vi "Main.vi"() -> ()   [LabVIEW 2014, in "Manipulator.lvclass"]
uses:
  Manipulator.lvclass
  typedefs/Coordinates.ctl
  <vilib>/Analysis/Matrix/Datatypes/RealMatrix.ctl
  typedefs/CommandStructure.ctl
  <vilib>/Analysis/Matrix/NI_Matrix.lvlib
panel:
  in  "STOP":bool
  out "Message":string
  in  "Visualization":refnum<k7>(container) caption="Visualisation in 3D"
  in  "Tab":enum32{"Visualisation 3D", "Trajectory Builder"}(tab)
  in  "MethodOfCalculation":u16(ring) items=["Geometric Method", "Denavit-Hartenberg Convention"]
  in  "AddPoint":bool
  in  "Cluster":T1={"Theta 1 "=45.0, "Theta 2"=90.0, "Theta 3"=90.0, "Theta 4"=90.0} {"Theta 4" min=0.0 max=180.0 step=0.5; "Theta 3" min=0.0 max=180.0 step=0.5; "Theta 2" min=0.0 max=180.0 step=0.5; "Theta 1" min=0.0 max=90.0 step=0.5}
  in  "CoordinatesIN":T2={"X"=141.5, "Y"=141.5, "Z"=220.5} {"X" step=0.5; "Y" step=0.5; "Z" step=0.5}
  out "ArrayOfNames\nOfPoints":string[](array[string])=["Point 1"]
  in  "NumberOfPoints":dbl=1.0 min=1.0 max=10.0 step=1.0
  in  "MatrixOfPoints":T3
  in  "Generate":bool
  # "CARTESIAN"
  # "JOINTS"
  # "PLEASE CHOOSE HOW MANY POINTS \nYOU WANT IN YOUR PATH"
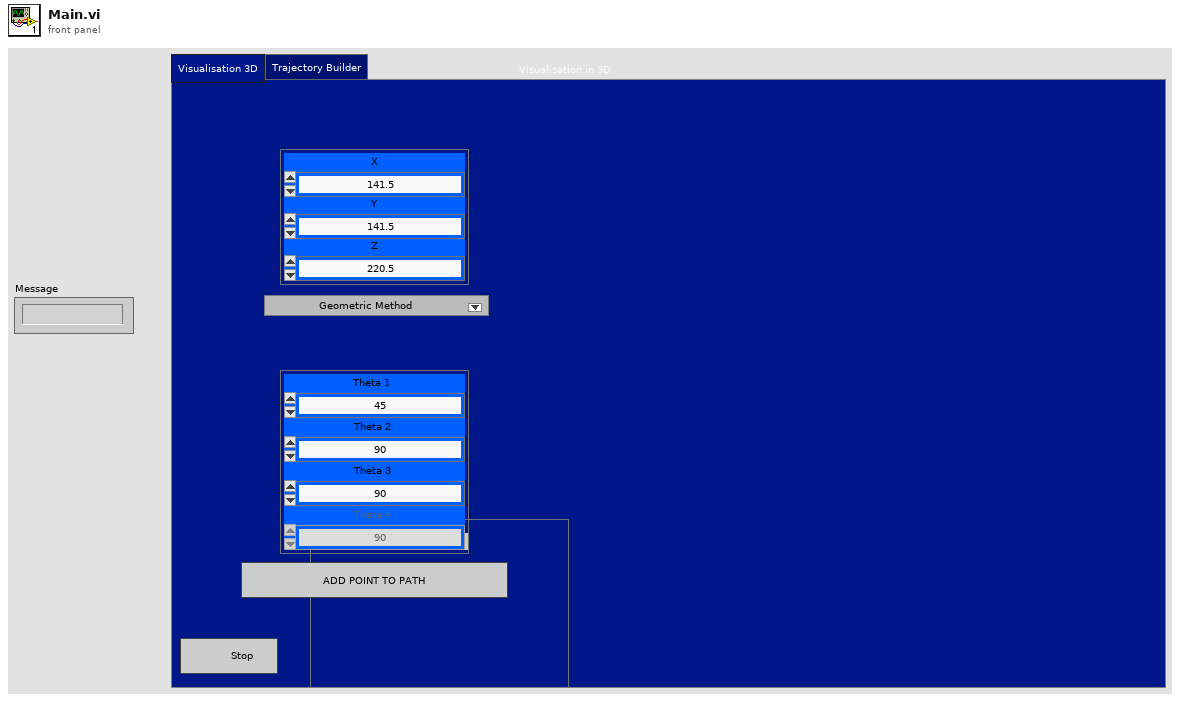
[diagram p1: front panel]
types:
  T1 = cluster{"Theta 1 ":dbl, "Theta 2":dbl, "Theta 3":dbl, "Theta 4":dbl}
  T2 = typedef "Manipulator.lvclass/Coordinates.ctl" = cluster{"X":dbl, "Y":dbl, "Z":dbl}
  T3 = typedef "NI_Matrix.lvlib/RealMatrix.ctl" = dbl[][]
  T4 = typedef "Manipulator.lvclass/CommandStructure.ctl" = cluster{"Command":string, "Data":variant}
  T5 = cluster{"Cluster":cluster{"Theta 1 ":dbl, "Theta 2":dbl, "Theta 3":dbl, "Theta 4":dbl}, "Cluster 2":cluster{"Theta 1 ":dbl, "Theta 2":dbl, "Theta 3":dbl, "Theta 4":dbl}}
  T6 = cluster{"NewVal":cluster{"X":dbl, "Y":dbl, "Z":dbl}, "OldVal":cluster{"X":dbl, "Y":dbl, "Z":dbl}}
  T7 = cluster{"Theta 1 ":dbl, "Theta 2":dbl, "Theta 3":dbl}
  T8 = cluster{"Numeric Control":dbl, "Numeric Control":dbl, "Numeric Control":dbl}
  T9 = cluster{"THETA_1":dbl, "THETA_2":dbl, "THETA_3":dbl, "THETA_4":dbl, "THETA_5":dbl, "THETA_6":dbl, "THETA_7":dbl, "THETA_8":dbl, "THETA_9":dbl, "THETA_10":dbl}[]
  T10 = cluster{"THETA_1":dbl, "THETA_2":dbl, "THETA_3":dbl, "THETA_4":dbl, "THETA_5":dbl, "THETA_6":dbl, "THETA_7":dbl, "THETA_8":dbl, "THETA_9":dbl, "THETA_10":dbl}
  T11 = cluster{"THETA_1":dbl, "THETA_2":dbl, "THETA_6":dbl, "THETA_4":dbl}
  T12 = cluster{"Numeric Control":dbl, "Numeric Control":dbl, "Numeric Control":dbl, "Numeric Control":dbl}
  T13 = cluster{"THETA_1":dbl, "THETA_2":dbl, "THETA_6":dbl, "THETA_4":dbl}[]
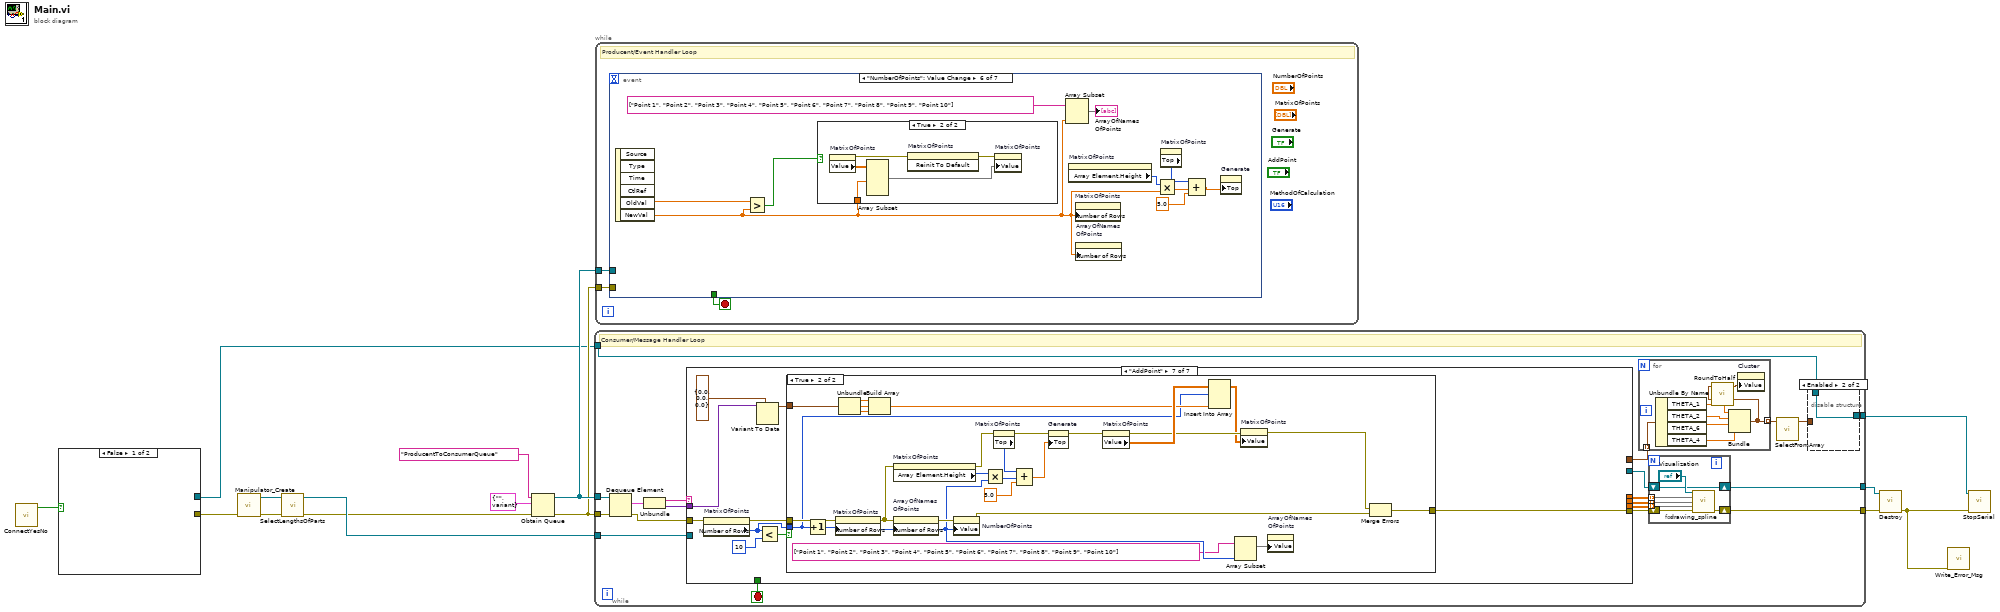
[diagram p0: block diagram]
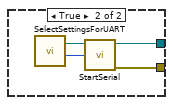
[diagram p2: hidden frame]
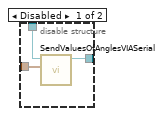
[diagram p3: hidden frame]
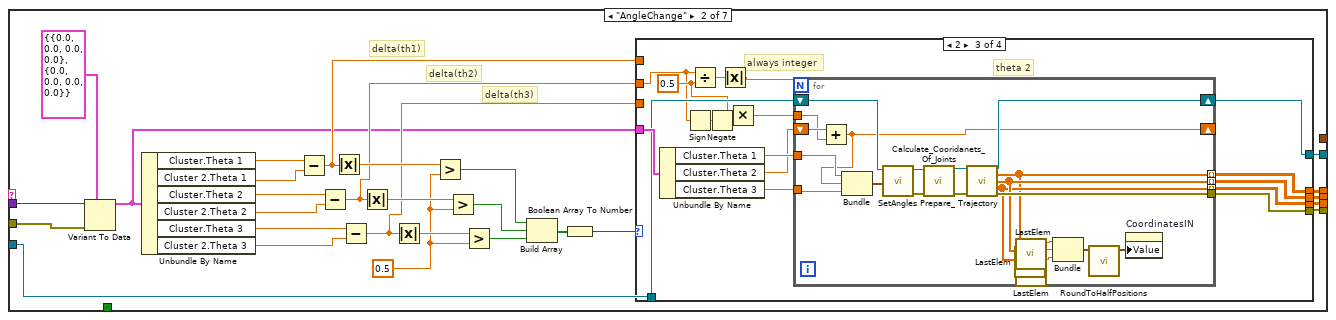
[diagram p5: hidden frame]
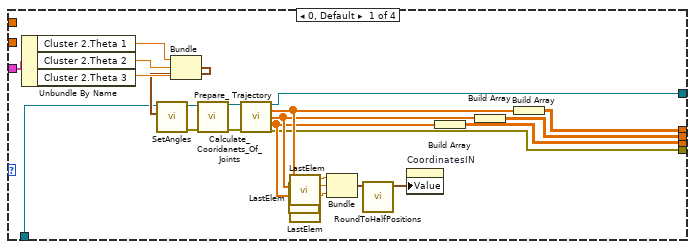
[diagram p6: hidden frame]
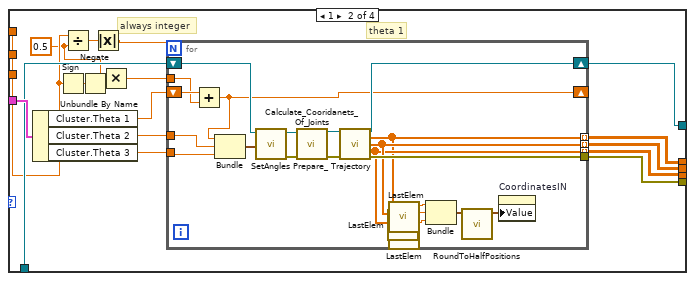
[diagram p7: hidden frame]
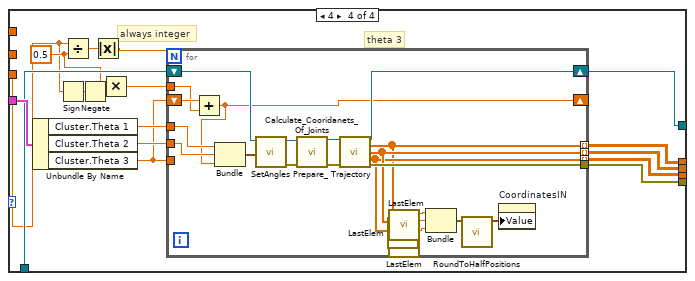
[diagram p8: hidden frame]
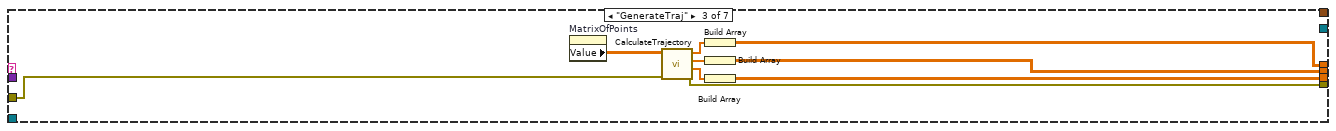
[diagram p9: hidden frame]
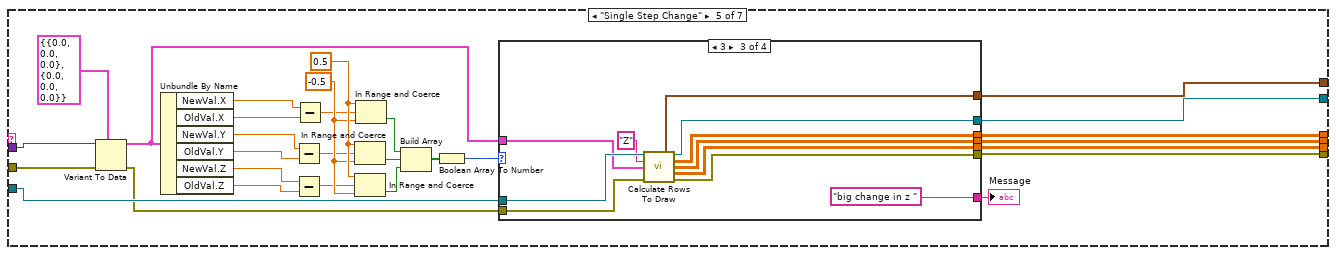
[diagram p11: hidden frame]
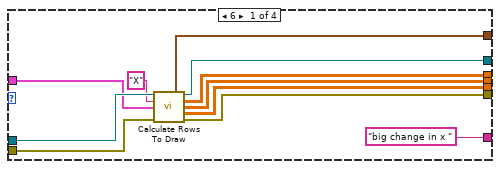
[diagram p12: hidden frame]
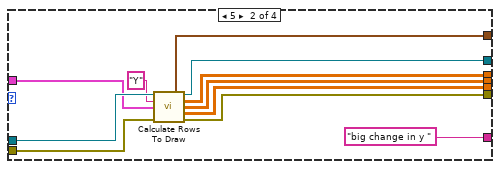
[diagram p13: hidden frame]
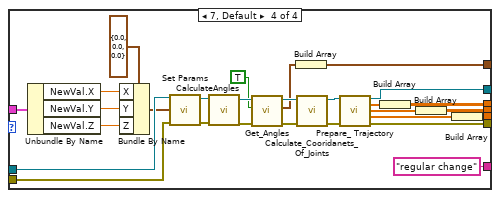
[diagram p14: hidden frame]
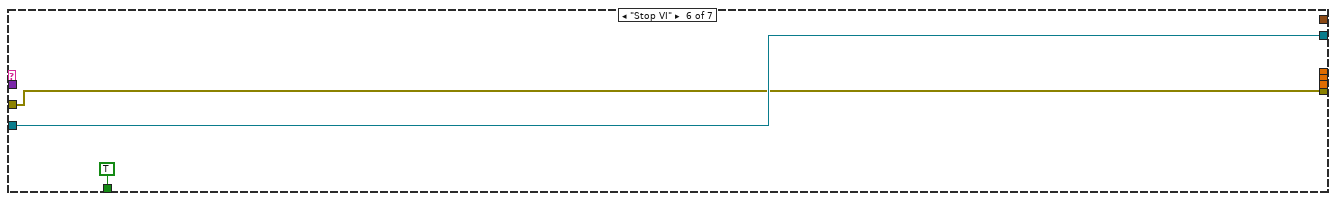
[diagram p15: hidden frame]
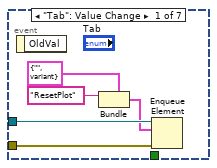
[diagram p17: hidden frame]
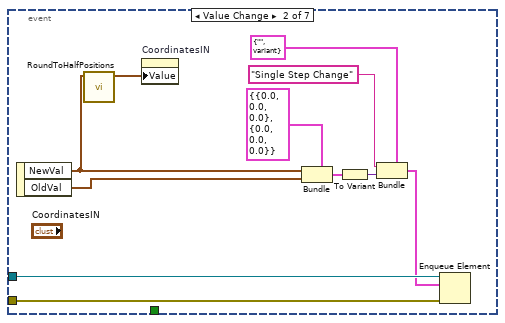
[diagram p18: hidden frame]
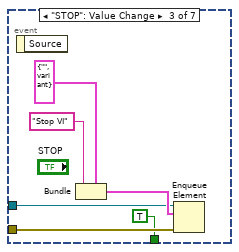
[diagram p19: hidden frame]
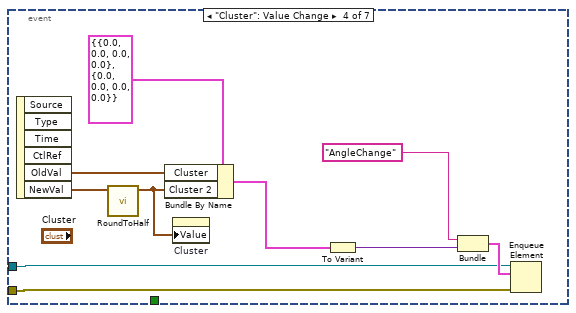
[diagram p20: hidden frame]
diagram:
  n1 = call "ConnectYesNo"() -> ("connect?"=w1:bool)  [unwired: 11 in]
  n2 = case shown="False" w1 {
    tunnel: [_ w19] -> w5
    tunnel: [_ w18] -> w4
    frame False {
    }
    frame True {
      n3 = call "SelectSettingsForUART.vi"() -> ("BaundRate"=w16:u32, "COMPort"=w17:refnum<visa-resource-name>)  [unwired: 10 in]
      n4 = call "StartSerial.vi"("baud rate"=w16, "VISA Refnum in"=w17) -> ("error out"=w19:errorcluster, "VISA Refnum out"=w18:refnum<visa-resource-name>)  [unwired: 8 in]
    }
  }
  n5 = call "Manipulator_Create.vi"("error in (no error)"=w5) -> ("error out"=w10:errorcluster, "reference out"=w12:refnum<class "Manipulator.lvclass">)  [unwired: 9 in]
  n6 = call-dynamic "SelectLengthsOfParts.vi"("error in (no error)"=w10, "reference in"=w12) -> ("error out"=w9:errorcluster, "reference out"=w11:refnum<class "Manipulator.lvclass">)  [unwired: 8 in]
  n7 = Obtain Queue(name (unnamed)="ProducentToConsumerQueue", element data type=T4 {"Command"="", "Data"=variant}, error in (no error)=w9) -> (queue out=w15:refnum<queue>, error out=w14:errorcluster)  [unwired: 2 in, 1 out]
  n8 = while {
    tunnel: w15 -> [w39]
    tunnel: w14 -> [w38]
    tunnel: w11 -> [w33]
    tunnel: [w30] -> w13
    tunnel: [w31] -> w6
    tunnel: w4 -> [w23]
    tunnel: [w22] -> w3
    stop <- w32 stop-if-true
    # "Consumer/Message Handler Loop"
    n9 = Dequeue Element(queue=w39, error in (no error)=w38) -> (element=w37:T4, error out=w34:errorcluster)  [unwired: 1 in, 2 out]
    n10 = Unbundle(w37) -> ("Command"=w36:string, "Data"=w35:variant)
    n11 = case shown="\"AddPoint\"" w36 {
      tunnel: w35 -> [_ w86 _ _ w260 _ w330]
      tunnel: [_ _ _ _ _ TRUE _] -> w32
      tunnel: w34 -> [w58 w85 w231 w233 w262 w324 w335]
      tunnel: w33 -> [_ w64 _ _ w242 w325 _]
      tunnel: [_ w63 _ _ w239 w325 _] -> w29
      tunnel: [w58 w62 w230 w233 w235 w324 w327] -> w28
      tunnel: [_ w61 w228 _ w238 _ _] -> w27
      tunnel: [_ w59 w226 _ w237 _ _] -> w26
      tunnel: [_ w60 w224 _ w236 _ _] -> w25
      tunnel: [_ _ _ _ w234 _ _] -> w24
      frame Default {
      }
      frame "AngleChange" {
        w75 = 0.5 ("y")
        # "delta(th3)"
        # "delta(th2)"
        # "delta(th1)"
        n12 = Variant To Data(error in=w85, type=T5 {"Cluster"={"Theta 1 "=0.0, "Theta 2"=0.0, "Theta 3"=0.0, "Theta 4"=0.0}, "Cluster 2"={"Theta 1 "=0.0, "Theta 2"=0.0, "Theta 3"=0.0, "Theta 4"=0.0}} ("input cluster"), Variant=w86) -> (data=w65:T5)  [unwired: 1 out]
        n13 = Unbundle By Name(w65) -> ("Cluster.Theta 1"=w66:dbl, "Cluster 2.Theta 1"=w83:dbl, "Cluster.Theta 2"=w82:dbl, "Cluster 2.Theta 2"=w81:dbl, "Cluster.Theta 3"=w80:dbl, "Cluster 2.Theta 3"=w79:dbl)
        n14 = Subtract(x=w66, y=w83) -> (x-y=w69:dbl)
        n15 = Subtract(x=w82, y=w81) -> (x-y=w67:dbl)
        n16 = Absolute Value(x=w69) -> (abs(x)=w78:dbl)
        n17 = Subtract(x=w80, y=w79) -> (x-y=w68:dbl)
        n18 = Absolute Value(x=w67) -> (abs(x)=w76:dbl)
        n19 = Absolute Value(x=w68) -> (abs(x)=w77:dbl)
        n20 = Greater?(x=w78, y=w75) -> (0:w74:bool)
        n21 = Greater?(x=w76, y=w75) -> (0:w73:bool)
        n22 = Greater?(x=w77, y=w75) -> (0:w72:bool)
        n23 = Build Array(w74, w73, w72) -> (w71:bool[])
        n24 = Boolean Array To Number(Boolean array=w71) -> (number=w70:u32)
        n25 = case shown="2" w70 {
          tunnel: w69 -> [_ w115 _ _]
          tunnel: w67 -> [_ _ w148 _]
          tunnel: w68 -> [_ _ _ w186]
          tunnel: w65 -> [w93 w126 w164 w202]
          tunnel: w64 -> [w88 w125 w163 w201]
          tunnel: [w87 w124 w162 w200] -> w63
          tunnel: [w94 w123 w161 w199] -> w62
          tunnel: [w99 w122 w160 w198] -> w61
          tunnel: [w95 w120 w158 w196] -> w60
          tunnel: [w97 w121 w159 w197] -> w59
          frame 0, Default {
            n26 = Unbundle By Name(w93) -> ("Cluster 2.Theta 1"=w92:dbl, "Cluster 2.Theta 2"=w91:dbl, "Cluster 2.Theta 3"=w90:dbl)
            n27 = Bundle("Theta 1"=w92, "Theta 2"=w91, "Theta 3"=w90) -> (w89:T7)  [unwired: 1 in]
            n28 = call-dynamic "SetAngles.vi"("Angles"=w89, "reference in"=w88) -> ("error out"=w106:errorcluster, "reference out"=w107:refnum<class "Manipulator.lvclass">)  [unwired: 8 in]
            n29 = call-dynamic "Calculate_Cooridanets_Of_Joints.vi"("error in (no error)"=w106, "reference in"=w107) -> ("error out"=w108:errorcluster, "reference out"=w109:refnum<class "Manipulator.lvclass">)  [unwired: 8 in]
            n30 = call-dynamic "Prepare_ Trajectory.vi"("reference in"=w109, "error in (no error)"=w108) -> ("reference out"=w87:refnum<class "Manipulator.lvclass">, "X"=w100:dbl[], "Y"=w98:dbl[], "Z"=w96:dbl[], "error out"=w94:errorcluster)  [unwired: 9 in]
            n31 = call "LastElem.vi"("X"=w98) -> ("Numeric Control"=w104:dbl)  [unwired: 10 in]
            n32 = call "LastElem.vi"("X"=w100) -> ("Numeric Control"=w105:dbl)  [unwired: 10 in]
            n33 = call "LastElem.vi"("X"=w96) -> ("Numeric Control"=w103:dbl)  [unwired: 10 in]
            n34 = Bundle("Numeric Control"=w105, "Numeric Control"=w104, "Numeric Control"=w103) -> (w102:T8)  [unwired: 1 in]
            n35 = call "RoundToHalfPositions.vi"("input cluster"=w102) -> ("output cluster"=w101:T8)  [unwired: 10 in]
            n36 = property on="CoordinatesIN" class="Clust (strict)"("Value"=w101) -> ()  [unwired: 2 in, 2 out]
            n37 = Build Array(w96) -> (w95:dbl[][])
            n38 = Build Array(w98) -> (w97:dbl[][])
            n39 = Build Array(w100) -> (w99:dbl[][])
          }
          frame 1 {
            w113 = 0.5 ("y")
            # "always integer"
            # "theta 1"
            n40 = Unbundle By Name(w126) -> ("Cluster.Theta 1"=w119:dbl, "Cluster.Theta 2"=w118:dbl, "Cluster.Theta 3"=w117:dbl)
            n41 = Sign(1:w115) -> (0:w114:dbl)
            n42 = Divide(x=w115, y=w113) -> (x/y=w116:dbl)
            n43 = Negate(x=w114) -> (-x=w111:dbl)
            n44 = Absolute Value(x=w116) -> (abs(x)=w110:dbl)
            n45 = Multiply(x=w113, y=w111) -> (x*y=w112:dbl)
            n46 = for {
              N: w110 -> [_]
              tunnel: [w132] -> w122 mode=indexing
              tunnel: [w134] -> w121 mode=indexing
              tunnel: [w133] -> w120 mode=indexing
              tunnel: [w141] -> w123
              shift-right: [w142] -> w124
              shift-left: w125 -> [w145]
              tunnel: w118 -> [w139]
              tunnel: w117 -> [w138]
              shift-right: [w135] -> _
              shift-left: w119 -> [w137]
              tunnel: w112 -> [w136]
              n47 = Add(x=w137, y=w136) -> (x+y=w135:dbl)
              n48 = Bundle(w135, "Theta 2"=w139, "Theta 3"=w138) -> (w140:cluster{dbl, "Theta 2":dbl, "Theta 3":dbl})  [unwired: 1 in]
              n49 = call-dynamic "SetAngles.vi"("Angles"=w140, "reference in"=w145) -> ("error out"=w143:errorcluster, "reference out"=w144:refnum<class "Manipulator.lvclass">)  [unwired: 8 in]
              n50 = call-dynamic "Calculate_Cooridanets_Of_Joints.vi"("error in (no error)"=w143, "reference in"=w144) -> ("error out"=w146:errorcluster, "reference out"=w147:refnum<class "Manipulator.lvclass">)  [unwired: 8 in]
              n51 = call-dynamic "Prepare_ Trajectory.vi"("reference in"=w147, "error in (no error)"=w146) -> ("reference out"=w142:refnum<class "Manipulator.lvclass">, "X"=w132:dbl[], "Y"=w134:dbl[], "Z"=w133:dbl[], "error out"=w141:errorcluster)  [unwired: 9 in]
              n52 = call "LastElem.vi"("X"=w134) -> ("Numeric Control"=w130:dbl)  [unwired: 10 in]
              n53 = call "LastElem.vi"("X"=w132) -> ("Numeric Control"=w131:dbl)  [unwired: 10 in]
              n54 = call "LastElem.vi"("X"=w133) -> ("Numeric Control"=w129:dbl)  [unwired: 10 in]
              n55 = Bundle("Numeric Control"=w131, "Numeric Control"=w130, "Numeric Control"=w129) -> (w128:T8)  [unwired: 1 in]
              n56 = call "RoundToHalfPositions.vi"("input cluster"=w128) -> ("output cluster"=w127:T8)  [unwired: 10 in]
              n57 = property on="CoordinatesIN" class="Clust (strict)"("Value"=w127) -> ()  [unwired: 2 in, 2 out]
            }
          }
          frame 2 {
            w154 = 0.5 ("y")
            # "always integer"
            # "theta 2"
            n58 = Unbundle By Name(w164) -> ("Cluster.Theta 1"=w150:dbl, "Cluster.Theta 2"=w149:dbl, "Cluster.Theta 3"=w157:dbl)
            n59 = Sign(1:w148) -> (0:w155:dbl)
            n60 = Divide(x=w148, y=w154) -> (x/y=w156:dbl)
            n61 = Negate(x=w155) -> (-x=w152:dbl)
            n62 = Absolute Value(x=w156) -> (abs(x)=w151:dbl)
            n63 = Multiply(x=w154, y=w152) -> (x*y=w153:dbl)
            n64 = for {
              N: w151 -> [_]
              tunnel: [w172] -> w160 mode=indexing
              tunnel: [w174] -> w159 mode=indexing
              tunnel: [w173] -> w158 mode=indexing
              tunnel: [w179] -> w161
              shift-right: [w180] -> w162
              shift-left: w163 -> [w183]
              tunnel: w157 -> [w177]
              shift-right: [w165] -> _
              shift-left: w149 -> [w176]
              tunnel: w153 -> [w175]
              tunnel: w150 -> [w166]
              n65 = Add(x=w176, y=w175) -> (x+y=w165:dbl)
              n66 = Bundle("Theta 1"=w166, w165, "Theta 3"=w177) -> (w178:cluster{"Theta 1 ":dbl, dbl, "Theta 3":dbl})  [unwired: 1 in]
              n67 = call-dynamic "SetAngles.vi"("Angles"=w178, "reference in"=w183) -> ("error out"=w181:errorcluster, "reference out"=w182:refnum<class "Manipulator.lvclass">)  [unwired: 8 in]
              n68 = call-dynamic "Calculate_Cooridanets_Of_Joints.vi"("error in (no error)"=w181, "reference in"=w182) -> ("error out"=w184:errorcluster, "reference out"=w185:refnum<class "Manipulator.lvclass">)  [unwired: 8 in]
              n69 = call-dynamic "Prepare_ Trajectory.vi"("reference in"=w185, "error in (no error)"=w184) -> ("reference out"=w180:refnum<class "Manipulator.lvclass">, "X"=w172:dbl[], "Y"=w174:dbl[], "Z"=w173:dbl[], "error out"=w179:errorcluster)  [unwired: 9 in]
              n70 = call "LastElem.vi"("X"=w174) -> ("Numeric Control"=w170:dbl)  [unwired: 10 in]
              n71 = call "LastElem.vi"("X"=w172) -> ("Numeric Control"=w171:dbl)  [unwired: 10 in]
              n72 = call "LastElem.vi"("X"=w173) -> ("Numeric Control"=w169:dbl)  [unwired: 10 in]
              n73 = Bundle("Numeric Control"=w171, "Numeric Control"=w170, "Numeric Control"=w169) -> (w168:T8)  [unwired: 1 in]
              n74 = call "RoundToHalfPositions.vi"("input cluster"=w168) -> ("output cluster"=w167:T8)  [unwired: 10 in]
              n75 = property on="CoordinatesIN" class="Clust (strict)"("Value"=w167) -> ()  [unwired: 2 in, 2 out]
            }
          }
          frame 4 {
            w193 = 0.5 ("y")
            # "always integer"
            # "theta 3"
            n76 = Unbundle By Name(w202) -> ("Cluster.Theta 1"=w189:dbl, "Cluster.Theta 2"=w188:dbl, "Cluster.Theta 3"=w187:dbl)
            n77 = Sign(1:w186) -> (0:w194:dbl)
            n78 = Divide(x=w186, y=w193) -> (x/y=w195:dbl)
            n79 = Negate(x=w194) -> (-x=w191:dbl)
            n80 = Absolute Value(x=w195) -> (abs(x)=w190:dbl)
            n81 = Multiply(x=w193, y=w191) -> (x*y=w192:dbl)
            n82 = for {
              N: w190 -> [_]
              tunnel: [w211] -> w198 mode=indexing
              tunnel: [w213] -> w197 mode=indexing
              tunnel: [w212] -> w196 mode=indexing
              tunnel: [w217] -> w199
              shift-right: [w218] -> w200
              shift-left: w201 -> [w221]
              tunnel: w188 -> [w205]
              tunnel: w187 -> [_]
              shift-right: [w203] -> _
              shift-left: w187 -> [w215]
              tunnel: w192 -> [w214]
              tunnel: w189 -> [w204]
              n83 = Add(x=w215, y=w214) -> (x+y=w203:dbl)
              n84 = Bundle("Theta 1"=w204, "Theta 2"=w205, w203) -> (w216:cluster{"Theta 1 ":dbl, "Theta 2":dbl, dbl})  [unwired: 1 in]
              n85 = call-dynamic "SetAngles.vi"("Angles"=w216, "reference in"=w221) -> ("error out"=w219:errorcluster, "reference out"=w220:refnum<class "Manipulator.lvclass">)  [unwired: 8 in]
              n86 = call-dynamic "Calculate_Cooridanets_Of_Joints.vi"("error in (no error)"=w219, "reference in"=w220) -> ("error out"=w222:errorcluster, "reference out"=w223:refnum<class "Manipulator.lvclass">)  [unwired: 8 in]
              n87 = call-dynamic "Prepare_ Trajectory.vi"("reference in"=w223, "error in (no error)"=w222) -> ("reference out"=w218:refnum<class "Manipulator.lvclass">, "X"=w211:dbl[], "Y"=w213:dbl[], "Z"=w212:dbl[], "error out"=w217:errorcluster)  [unwired: 9 in]
              n88 = call "LastElem.vi"("X"=w213) -> ("Numeric Control"=w209:dbl)  [unwired: 10 in]
              n89 = call "LastElem.vi"("X"=w211) -> ("Numeric Control"=w210:dbl)  [unwired: 10 in]
              n90 = call "LastElem.vi"("X"=w212) -> ("Numeric Control"=w208:dbl)  [unwired: 10 in]
              n91 = Bundle("Numeric Control"=w210, "Numeric Control"=w209, "Numeric Control"=w208) -> (w207:T8)  [unwired: 1 in]
              n92 = call "RoundToHalfPositions.vi"("input cluster"=w207) -> ("output cluster"=w206:T8)  [unwired: 10 in]
              n93 = property on="CoordinatesIN" class="Clust (strict)"("Value"=w206) -> ()  [unwired: 2 in, 2 out]
            }
          }
        }
      }
      frame "GenerateTraj" {
        n94 = property on="MatrixOfPoints" class="Arr (strict)"() -> ("Value"=w232:T3)  [unwired: 2 in, 2 out]
        n95 = call "CalculateTrajectory.vi"("error in (no error)"=w231, "MatrixOfPoints"=w232) -> ("error out"=w230:errorcluster, "z"=w225:dbl[], "y"=w227:dbl[], "x"=w229:dbl[])  [unwired: 6 in]
        n96 = Build Array(w229) -> (w228:dbl[][])
        n97 = Build Array(w227) -> (w226:dbl[][])
        n98 = Build Array(w225) -> (w224:dbl[][])
      }
      frame "ResetPlot" {
      }
      frame "Single Step Change" {
        w258 = -0.5 ("lower limit")
        w259 = 0.5 ("upper limit")
        n99 = Variant To Data(error in=w262, type=T6 {"NewVal"={"X"=0.0, "Y"=0.0, "Z"=0.0}, "OldVal"={"X"=0.0, "Y"=0.0, "Z"=0.0}}, Variant=w260) -> (data=w240:T6, error out=w241:errorcluster)
        n100 = Unbundle By Name(w240) -> ("NewVal.X"=w254:dbl, "OldVal.X"=w253:dbl, "NewVal.Y"=w252:dbl, "OldVal.Y"=w251:dbl, "NewVal.Z"=w250:dbl, "OldVal.Z"=w249:dbl)
        n101 = Subtract(x=w252, y=w251) -> (x-y=w256:dbl)
        n102 = Subtract(x=w250, y=w249) -> (x-y=w255:dbl)
        n103 = Subtract(x=w254, y=w253) -> (x-y=w257:dbl)
        n104 = In Range and Coerce(upper limit=w259, x=w256, lower limit=w258) -> (In Range?=w247:bool)  [unwired: 1 out]
        n105 = In Range and Coerce(upper limit=w259, x=w255, lower limit=w258) -> (In Range?=w246:bool)  [unwired: 1 out]
        n106 = In Range and Coerce(upper limit=w259, x=w257, lower limit=w258) -> (In Range?=w248:bool)  [unwired: 1 out]
        n107 = Build Array(w248, w247, w246) -> (w245:bool[])
        n108 = Boolean Array To Number(Boolean array=w245) -> (number=w244:u32)
        n109 = case shown="3" w244 {
          tunnel: ["big change in x " "big change in y " "big change in z " "regular change"] -> w243
          tunnel: w242 -> [w272 w283 w294 w318]
          tunnel: w240 -> [w270 w281 w292 w323]
          tunnel: w241 -> [w271 w282 w293 w319]
          tunnel: [w267 w278 w289 w312] -> w239
          tunnel: [w266 w277 w288 w301] -> w238
          tunnel: [w265 w276 w287 w300] -> w237
          tunnel: [w264 w275 w286 w299] -> w236
          tunnel: [w268 w279 w290 w302] -> w235
          tunnel: [w263 w274 w285 w296] -> w234
          frame 6 {
            n110 = call "Calculate Rows To Draw.vi"("reference in"=w272, "WhichAxis?"="X", "InData"=w270, "error in (no error)"=w271) -> ("ArrayOfAngles"=w263:T9, "reference out"=w267:refnum<class "Manipulator.lvclass">, "X"=w266:dbl[][], "Y"=w265:dbl[][], "Z"=w264:dbl[][], "error out"=w268:errorcluster)  [unwired: 6 in]
          }
          frame 5 {
            n111 = call "Calculate Rows To Draw.vi"("reference in"=w283, "WhichAxis?"="Y", "InData"=w281, "error in (no error)"=w282) -> ("ArrayOfAngles"=w274:T9, "reference out"=w278:refnum<class "Manipulator.lvclass">, "X"=w277:dbl[][], "Y"=w276:dbl[][], "Z"=w275:dbl[][], "error out"=w279:errorcluster)  [unwired: 6 in]
          }
          frame 3 {
            n112 = call "Calculate Rows To Draw.vi"("reference in"=w294, "WhichAxis?"="Z", "InData"=w292, "error in (no error)"=w293) -> ("ArrayOfAngles"=w285:T9, "reference out"=w289:refnum<class "Manipulator.lvclass">, "X"=w288:dbl[][], "Y"=w287:dbl[][], "Z"=w286:dbl[][], "error out"=w290:errorcluster)  [unwired: 6 in]
          }
          frame 7, Default {
            n113 = Unbundle By Name(w323) -> ("NewVal.X"=w322:dbl, "NewVal.Y"=w321:dbl, "NewVal.Z"=w320:dbl)
            n114 = Bundle By Name(cluster=T2 {"X"=0.0, "Y"=0.0, "Z"=0.0} ("CoordinatesIN"), "X"=w322, "Y"=w321, "Z"=w320) -> (w317:T2)
            n115 = call-dynamic "Set Params.vi"("error in (no error)"=w319, "CoordinatesIN"=w317, "reference in"=w318) -> ("error out"=w314:errorcluster, "reference out"=w313:refnum<class "Manipulator.lvclass">)  [unwired: 7 in]
            n116 = call "CalculateAngles.vi"("error in (no error)"=w314, "reference in"=w313) -> ("error out"=w307:errorcluster, "reference out"=w310:refnum<class "Manipulator.lvclass">)  [unwired: 8 in]
            n117 = call-dynamic "Get_Angles.vi"("error in (no error)"=w307, "Deg?"=TRUE, "reference in"=w310) -> ("error out"=w308:errorcluster, "Angles"=w297:T10, "reference out"=w309:refnum<class "Manipulator.lvclass">)  [unwired: 6 in]
            n118 = Build Array(w297) -> (w296:T9)
            n119 = call-dynamic "Calculate_Cooridanets_Of_Joints.vi"("error in (no error)"=w308, "reference in"=w309) -> ("error out"=w315:errorcluster, "reference out"=w316:refnum<class "Manipulator.lvclass">)  [unwired: 8 in]
            n120 = call-dynamic "Prepare_ Trajectory.vi"("reference in"=w316, "error in (no error)"=w315) -> ("reference out"=w312:refnum<class "Manipulator.lvclass">, "X"=w305:dbl[], "Y"=w304:dbl[], "Z"=w303:dbl[], "error out"=w302:errorcluster)  [unwired: 9 in]
            n121 = Build Array(w305) -> (w301:dbl[][])
            n122 = Build Array(w304) -> (w300:dbl[][])
            n123 = Build Array(w303) -> (w299:dbl[][])
          }
        }
        "Message" <- w243
      }
      frame "Stop VI" {
      }
      frame "AddPoint" {
        n124 = property on="MatrixOfPoints" class="Arr (strict)"(error in=w335) -> (error out=w328:errorcluster, "Number of Rows"=w332:u32)  [unwired: 1 in, 1 out]
        n125 = Variant To Data(type=T2 {"X"=0.0, "Y"=0.0, "Z"=0.0} ("CoordinatesIN"), Variant=w330) -> (data=w331:T2)  [unwired: 1 in, 1 out]
        n126 = Less?(x=w332, y=u32 10) -> (x < y?=w333:bool)
        n127 = case shown="True" w333 {
          tunnel: w328 -> [_ w347]
          tunnel: w332 -> [_ w342]
          tunnel: w331 -> [_ w352]
          tunnel: [_ w339] -> w327
          frame False {
          }
          frame True {
            n128 = Increment(x=w342) -> (x+1=w338:u32)
            n129 = property on="MatrixOfPoints" class="Arr (strict)"(error in=w347, "Number of Rows"=w338) -> (error out=w361:errorcluster)  [unwired: 1 in, 1 out]
            n130 = Unbundle(w352) -> ("X"=w349:dbl, "Y"=w350:dbl, "Z"=w351:dbl)
            n131 = Build Array(w349, w350, w351) -> (w345:dbl[])
            n132 = property on="MatrixOfPoints" class="Arr (strict)"(error in=w361) -> (error out=w355:errorcluster, "Array Element.Height"=w356:u32)  [unwired: 1 in, 1 out]
            n133 = property on="ArrayOfNames\nOfPoints" class="Arr (strict)"(error in=w361, "Number of Rows"=w338) -> (error out=w353:errorcluster)  [unwired: 1 in, 1 out]
            n134 = property on="NumberOfPoints" class="DigNum (strict)"(error in=w353, "Value"=w338) -> (error out=w348:errorcluster)  [unwired: 1 in, 1 out]
            n135 = Multiply(x=w356, y=w338) -> (x*y=w359:u32)
            n136 = property on="MatrixOfPoints" class="Arr (strict)"(error in=w355) -> (error out=w354:errorcluster, "Top"=w358:i32)  [unwired: 1 in, 1 out]
            n137 = Compound Arithmetic op=unknown(w358, w359, 5.0 ("y")) -> (w357:dbl)
            n138 = property on="Generate" class="Bool"(error in=w354, "Top"=w357) -> (error out=w341:errorcluster)  [unwired: 1 in, 1 out]
            n139 = property on="MatrixOfPoints" class="Arr (strict)"(error in=w341) -> (error out=w344:errorcluster, "Value"=w346:dbl[][])  [unwired: 1 in, 1 out]
            n140 = Insert Into Array(array=w346, index (row)=w342, new element=w345) -> (w343:dbl[][])  [unwired: 1 in]
            n141 = Array Subset(array=string[] ["Point 1", "Point 2", "Point 3", "Point 4", "Point 5", "Point 6", "Point 7", "Point 8", "Point 9", "Point 10"], length=w338) -> (w336:string[])  [unwired: 1 in]
            n142 = property on="MatrixOfPoints" class="Arr (strict)"(error in=w344, "Value"=w343) -> (error out=w340:errorcluster)  [unwired: 1 in, 1 out]
            n143 = property on="ArrayOfNames\nOfPoints" class="Arr (strict)"("Value"=w336) -> ()  [unwired: 2 in, 2 out]
            n144 = Merge Errors(w340, w348) -> (w339:errorcluster)
          }
        }
      }
    }
    n145 = for {
      tunnel: [w44] -> w21 mode=indexing
      tunnel: w24 -> [w45] mode=indexing
      n146 = Unbundle By Name(w45) -> ("THETA_1"=w50:dbl, "THETA_2"=w49:dbl, "THETA_6"=w48:dbl, "THETA_4"=w47:dbl)
      n147 = Bundle("THETA_1"=w50, "THETA_2"=w49, "THETA_6"=w48, "THETA_4"=w47) -> (w44:T11)  [unwired: 1 in]
      n148 = call "RoundToHalf.vi"("Cluster in"=w44) -> ("Cluster out"=w46:T12)  [unwired: 10 in]
      n149 = property on="Cluster" class="Clust (strict)"("Value"=w46) -> ()  [unwired: 2 in, 2 out]
    }
    n150 = for {
      tunnel: w26 -> [w56] mode=indexing
      tunnel: w25 -> [w55] mode=indexing
      shift-right: [w53] -> w30
      shift-left: w28 -> [w54]
      tunnel: w27 -> [w52] mode=indexing
      shift-right: [w51] -> w31
      shift-left: w29 -> [w51]
      n151 = call "drawing_spline.vi"("Automation Refnum in"="Visualization", "Wpó³rzêdne X"=w52, "Wspó³rzêdne Y"=w56, "Wspó³rzêdne Z"=w55, "error in (no error)"=w54) -> ("error out"=w53:errorcluster)  [unwired: 10 in]
    }
    n152 = call "SelectFromArray.vi"("Array in"=w21) -> ("Array out"=w20:T13)  [unwired: 10 in]
    n153 = disable-structure shown="Enabled" {
      disable-tunnel: w23 -> [w42 w43]
      disable-tunnel: [w41 w43] -> w22
      disable-tunnel: w20 -> [w40 _]
      frame Disabled {
        n154 = call "SendValuesOfAnglesVIASerial.vi"("Data"=w40, "VISA Refnum in"=w42) -> ("VISA Refnum out"=w41:refnum<visa-resource-name>)  [unwired: 8 in, 1 out]
      }
      frame Enabled {
      }
    }
  }
  n155 = while {
    tunnel: w15 -> [w364]
    tunnel: w14 -> [w363]
    stop <- w362 stop-if-true
    # "Producent/Event Handler Loop"
    n156 = event shown="[5] \"NumberOfPoints\": Value Change" {
      selector: _ -> [_ _ _ _ _ _ _]
      dyn-events: _ -> [_ _ _ _ _ _ _]
      timeout: _ -> [_ _ _ _ _ _ _]
      tunnel: w364 -> [w368 w376 w383 w394 w398 _ w422]
      tunnel: w363 -> [w369 w380 w382 w393 w397 _ w421]
      tunnel: [_ _ TRUE _ _ _ _] -> w362
      event "Tab": Value Change {
        n157 = event-data() -> ()  [unwired: 1 in, 1 out]
        n158 = Bundle(cluster=T4 {"Command"="", "Data"=variant}, "Command"="ResetPlot") -> (w366:T4)  [unwired: 1 in]
        n159 = Enqueue Element(queue=w368, element=w366, error in (no error)=w369) -> ()  [unwired: 1 in, 3 out]
      }
      event Value Change {
        n160 = event-data() -> ("NewVal"=w371:T2, "OldVal"=w378:T2)  [unwired: 1 in]
        n161 = call "RoundToHalfPositions.vi"("input cluster"=w371) -> ("output cluster"=w370:T8)  [unwired: 10 in]
        n162 = property on="CoordinatesIN" class="Clust (strict)"("Value"=w370) -> ()  [unwired: 2 in, 2 out]
        n163 = Bundle(cluster=T6 {"NewVal"={"X"=0.0, "Y"=0.0, "Z"=0.0}, "OldVal"={"X"=0.0, "Y"=0.0, "Z"=0.0}}, "NewVal"=w371, "OldVal"=w378) -> (w377:T6)
        n164 = To Variant(anything=w377) -> (Variant=w373:variant)
        n165 = Bundle(cluster=T4 {"Command"="", "Data"=variant}, "Command"="Single Step Change", "Data"=w373) -> (w372:T4)
        n166 = Enqueue Element(queue=w376, element=w372, error in (no error)=w380) -> ()  [unwired: 1 in, 3 out]
      }
      event "STOP": Value Change {
        n167 = event-data() -> ()  [unwired: 1 in, 1 out]
        n168 = Bundle(cluster=T4 {"Command"="", "Data"=variant}, "Command"="Stop VI") -> (w385:T4)  [unwired: 1 in]
        n169 = Enqueue Element(queue=w383, element=w385, error in (no error)=w382) -> ()  [unwired: 1 in, 3 out]
      }
      event "Cluster": Value Change {
        n170 = event-data() -> ("OldVal"=w392:T1, "NewVal"=w388:T1)  [unwired: 1 in, 4 out]
        n171 = call "RoundToHalf.vi"("Cluster in"=w388) -> ("Cluster out"=w387:T12)  [unwired: 10 in]
        n172 = Bundle By Name(cluster=T5 {"Cluster"={"Theta 1 "=0.0, "Theta 2"=0.0, "Theta 3"=0.0, "Theta 4"=0.0}, "Cluster 2"={"Theta 1 "=0.0, "Theta 2"=0.0, "Theta 3"=0.0, "Theta 4"=0.0}} ("input cluster"), "Cluster"=w392, "Cluster 2"=w387) -> (w390:T5)
        n173 = property on="Cluster" class="Clust (strict)"("Value"=w387) -> ()  [unwired: 2 in, 2 out]
        n174 = To Variant(anything=w390) -> (Variant=w391:variant)
        n175 = Bundle("AngleChange", "Variant"=w391) -> (w395:cluster{string, "Variant":variant})  [unwired: 1 in]
        n176 = Enqueue Element(queue=w394, element=w395, error in (no error)=w393) -> ()  [unwired: 1 in, 3 out]
      }
      event "AddPoint": Value Change {
        n177 = event-data() -> ("NewVal"=w399:bool)  [unwired: 1 in, 5 out]
        n178 = case shown="True" w399 {
          tunnel: w398 -> [_ w404]
          tunnel: w397 -> [_ w403]
          frame False {
          }
          frame True {
            n179 = property on="CoordinatesIN" class="Clust (strict)"() -> ("Value"=w401:T2)  [unwired: 2 in, 2 out]
            n180 = To Variant(anything=w401) -> (Variant=w402:variant)
            n181 = Bundle("AddPoint", "Variant"=w402) -> (w405:cluster{string, "Variant":variant})  [unwired: 1 in]
            n182 = Enqueue Element(queue=w404, element=w405, error in (no error)=w403) -> ()  [unwired: 1 in, 3 out]
          }
        }
      }
      event "NumberOfPoints": Value Change {
        n183 = event-data() -> ("OldVal"=w408:dbl, "NewVal"=w406:dbl)  [unwired: 1 in, 4 out]
        n184 = Greater?(x=w408, y=w406) -> (0:w407:bool)
        n185 = case shown="True" w407 {
          tunnel: w406 -> [_ w419]
          frame False {
          }
          frame True {
            n186 = property on="MatrixOfPoints" class="Arr (strict)"() -> (error out=w418:errorcluster, "Value"=w420:T3)  [unwired: 2 in, 1 out]
            n187 = Array Subset(array=w420, length (row)=w419) -> (w416:T3)  [unwired: 3 in]
            n188 = invoke on="MatrixOfPoints" class="Arr (strict)" method="Reinit To Default"(error in=w418) -> (error out=w417:errorcluster)  [unwired: 2 in, 2 out]
            n189 = property on="MatrixOfPoints" class="Arr (strict)"(error in=w417, "Value"=w416) -> ()  [unwired: 1 in, 2 out]
          }
        }
        n190 = Array Subset(array=string[] ["Point 1", "Point 2", "Point 3", "Point 4", "Point 5", "Point 6", "Point 7", "Point 8", "Point 9", "Point 10"], length=w406) -> (→"ArrayOfNames\nOfPoints":string[])  [unwired: 1 in]
        n191 = property on="MatrixOfPoints" class="Arr (strict)"() -> ("Array Element.Height"=w413:u32)  [unwired: 2 in, 2 out]
        n192 = property on="MatrixOfPoints" class="Arr (strict)"("Number of Rows"=w406) -> ()  [unwired: 2 in, 2 out]
        n193 = property on="ArrayOfNames\nOfPoints" class="Arr (strict)"("Number of Rows"=w406) -> ()  [unwired: 2 in, 2 out]
        n194 = Multiply(x=w413, y=w406) -> (x*y=w410:dbl)
        n195 = property on="MatrixOfPoints" class="Arr (strict)"() -> ("Top"=w411:i32)  [unwired: 2 in, 2 out]
        n196 = Compound Arithmetic op=ADD(w411, w410, 5.0 ("y")) -> (w412:dbl)
        n197 = property on="Generate" class="Bool"("Top"=w412) -> ()  [unwired: 2 in, 2 out]
      }
      event "Generate": Value Change {
        n198 = event-data() -> ("NewVal"=w423:bool)  [unwired: 1 in, 5 out]
        n199 = case shown="True" w423 {
          tunnel: w422 -> [_ w425]
          tunnel: w421 -> [_ w424]
          frame False {
          }
          frame True {
            n200 = Bundle(cluster=T4 {"Command"="", "Data"=variant}, "Command"="GenerateTraj") -> (w427:T4)  [unwired: 1 in]
            n201 = Enqueue Element(queue=w425, element=w427, error in (no error)=w424) -> ()  [unwired: 1 in, 3 out]
          }
        }
      }
    }
  }
  n202 = call-dynamic "Destroy.vi"("error in (no error)"=w13, "reference in"=w6) -> ("error out"=w2:errorcluster)  [unwired: 8 in, 1 out]
  n203 = call "Write_Error_Msg.vi"("error in (no error)"=w2) -> ()  [unwired: 10 in, 1 out]
  n204 = call "StopSerial.vi"("error in (no error)"=w2, "VISA Refnum in"=w3) -> ()  [unwired: 10 in]
